vi "ReleaseQueues.vi"(8 "error in (no error)":errorcluster, 11 "Generator":refnum<class "Generator.lvclass">) -> (0 "error out":errorcluster, 3 "Generator out":refnum<class "Generator.lvclass">)   [LabVIEW 2019, in "Generator.lvclass"]
uses:
  Generator.lvclass
  Generator.lvclass/Generator.ctl
panel:
  # "For instructions on how to use the JKI State Machine Objects, examples and video tutorials, visit:\nhttp://jki.net/state-machine-objects/\n\nJKI State Machine Objects™\nhttp://jki.net/state-machine-objects/\nCopyright (C) 2005-2015, JKI <info@jki.net>\nALL RIGHTS RESERVED"
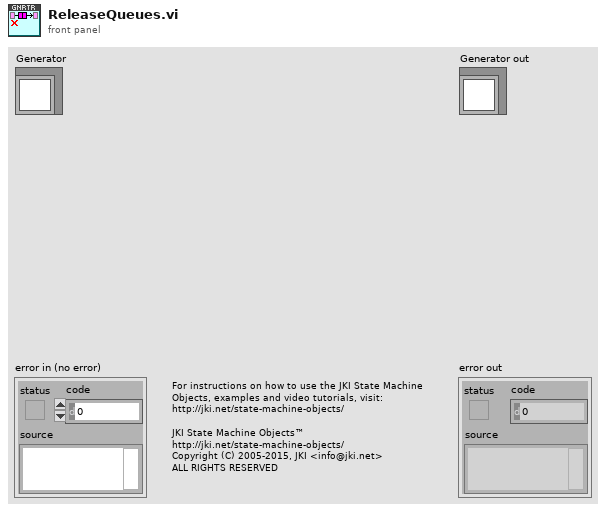
[diagram p1: front panel]
types:
  T1 = typedef "Generator.lvclass/PrivateQueues--Cluster.ctl" = cluster{"Message":refnum<queue>, "Sampling":refnum<queue>, "AOchannels":refnum<queue>, "REFchannels":refnum<queue>, "Sweep":refnum<queue>}
  T2 = typedef "Generator.lvclass/PublicQueues--Cluster.ctl" = cluster{"AOwfm":refnum<queue>}
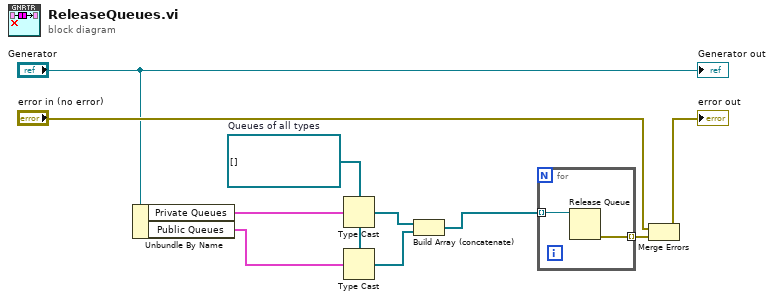
[diagram p0: block diagram]
diagram:
  w1 = refnum<queue>[] []  # Queues of all types
  n1 = Unbundle By Name("Generator") -> ("Private Queues"=w8:T1, "Public Queues"=w5:T2)
  n2 = Type Cast(type=w1, x=w8) -> (*(type *) &x=w3:refnum<queue>[])
  n3 = Type Cast(type=w1, x=w5) -> (*(type *) &x=w4:refnum<queue>[])
  n4 = Build Array (concatenate)(w3, w4) -> (w2:refnum<queue>[])
  n5 = for {
    tunnel: w2 -> [w11] mode=indexing
    tunnel: [w12] -> w10 mode=indexing
    n6 = Release Queue(queue=w11) -> (error out=w12:errorcluster)  [unwired: 2 in, 2 out]
  }
  n7 = Merge Errors("error in (no error)", w10) -> (→"error out":errorcluster)
  "Generator out" <- "Generator"
